vi "Convertor.vi"(11 "机器人指令数组":string[][](array[string])) -> (3 "机器人语音指令数据簇":T1)   [LabVIEW 2014, in "Voice.lvlib" / "Voice.lvclass"]
uses:
  Voice.lvclass
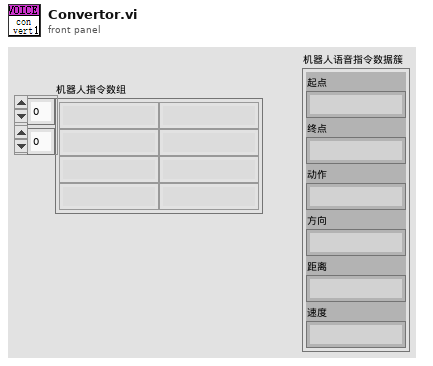
[diagram p1: front panel]
types:
  T1 = cluster{"起点":string, "终点":string, "动作":string, "方向":string, "距离":string, "速度":string}
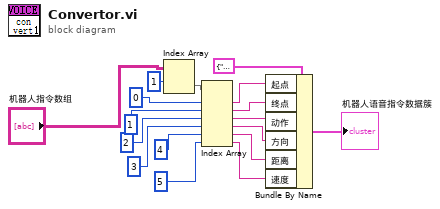
[diagram p0: block diagram]
diagram:
  n1 = Index Array(array="机器人指令数组", index (row)=1 ("索引 (行)")) -> (element=w3:string[])  [unwired: 1 in]
  n2 = Index Array(array=w3, index #1=0 ("索引"), index #2=1 ("索引"), index #3=2 ("索引"), index #4=3 ("索引"), index #5=4 ("索引"), index #6=5 ("索引")) -> (element #1=w11:string, element #2=w12:string, element #3=w13:string, element #4=w14:string, element #5=w15:string, element #6=w16:string)
  n3 = Bundle By Name(cluster=T1 {"起点"="", "终点"="", "动作"="", "方向"="", "距离"="", "速度"=""} ("VoiceControl_Cmd_Cluster"), "起点"=w11, "终点"=w12, "动作"=w13, "方向"=w14, "距离"=w15, "速度"=w16) -> (→"机器人语音指令数据簇":T1)
